vi "check mergeable.vi"(10 "Cube 2":T1, 11 "Cube 1":T1) -> (2 "Merged?":bool, 3 "Cube Out":T1)   [LabVIEW 2021]
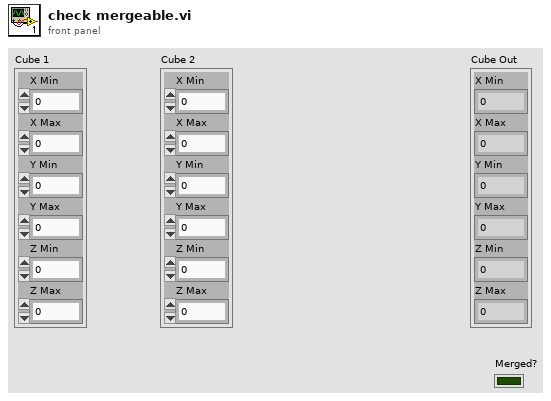
[diagram p1: front panel]
types:
  T1 = cluster{"X Min":i64, "X Max":i64, "Y Min":i64, "Y Max":i64, "Z Min":i64, "Z Max":i64}
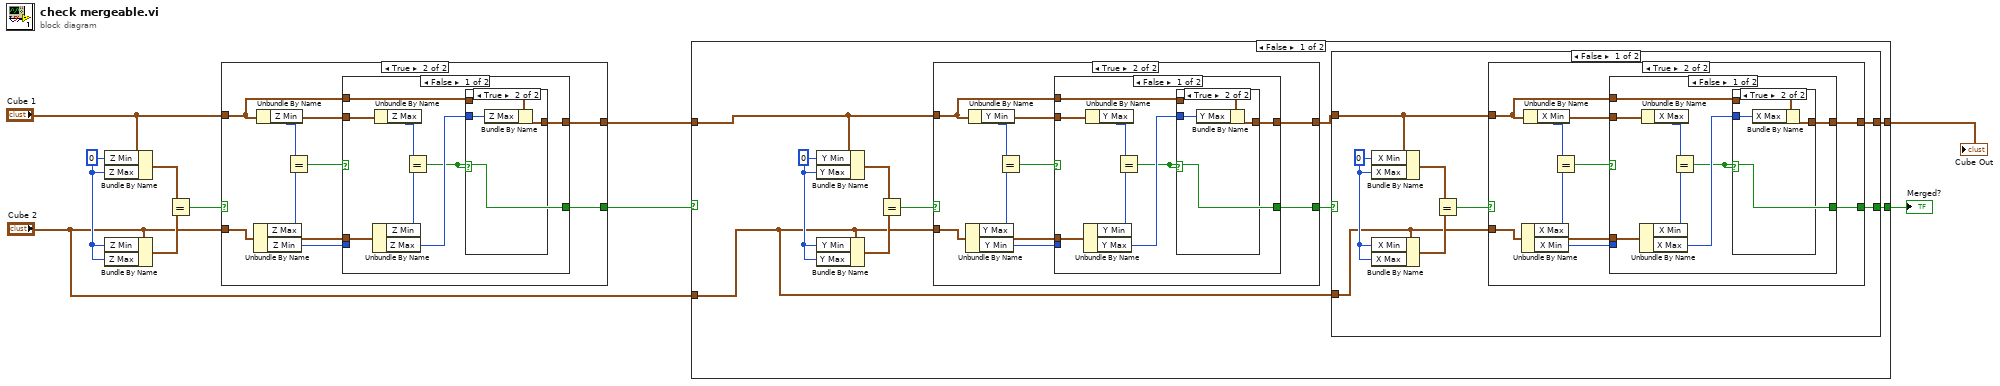
[diagram p0: block diagram]
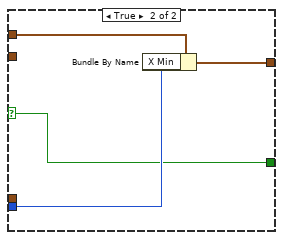
[diagram p4: hidden frame]
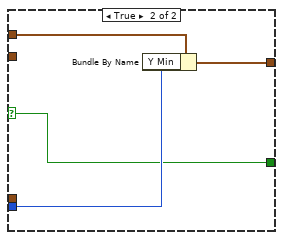
[diagram p8: hidden frame]
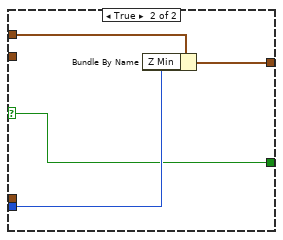
[diagram p12: hidden frame]
diagram:
  w10 = i64 0 ("Z Min")
  n1 = Bundle By Name(cluster="Cube 1", "Z Min"=w10, "Z Max"=w10) -> (w8:T1)
  n2 = Bundle By Name(cluster="Cube 2", "Z Min"=w10, "Z Max"=w10) -> (w9:T1)
  n3 = Equal?(x=w8, y=w9) -> (x = y?=w7:bool)
  n4 = case shown="True" w7 {
    selector: w7 -> [w12 _]
    tunnel: [w12 w15] -> w2
    tunnel: "Cube 1" -> [w11 w13]
    tunnel: "Cube 2" -> [_ w14]
    tunnel: [w11 w17] -> w5
    frame False {
    }
    frame True {
      n5 = Unbundle By Name(w14) -> ("Z Max"=w19:i64, "Z Min"=w18:i64)
      n6 = Unbundle By Name(w13) -> ("Z Min"=w20:i64)
      n7 = Equal?(x=w20, y=w19) -> (x = y?=w16:bool)
      n8 = case shown="False" w16 {
        selector: w16 -> [_ w33]
        tunnel: w13 -> [w24 w36]
        tunnel: w18 -> [_ w35]
        tunnel: [w22 w34] -> w17
        tunnel: [w21 w33] -> w15
        tunnel: w14 -> [w26 _]
        tunnel: w13 -> [w25 _]
        frame False {
          n9 = Unbundle By Name(w26) -> ("Z Min"=w28:i64, "Z Max"=w23:i64)
          n10 = Unbundle By Name(w25) -> ("Z Max"=w27:i64)
          n11 = Equal?(x=w27, y=w28) -> (x = y?=w21:bool)
          n12 = case shown="True" w21 {
            tunnel: w24 -> [w29 w32]
            tunnel: w23 -> [_ w31]
            tunnel: [w29 w30] -> w22
            frame False {
            }
            frame True {
              n13 = Bundle By Name(cluster=w32, "Z Max"=w31) -> (w30:T1)
            }
          }
        }
        frame True {
          n14 = Bundle By Name(cluster=w36, "Z Min"=w35) -> (w34:T1)
        }
      }
    }
  }
  n15 = case shown="False" w2 {
    selector: w2 -> [_ w110]
    tunnel: w5 -> [w42 w109]
    tunnel: "Cube 2" -> [w41 _]
    tunnel: [w39 w110] -> w3
    tunnel: [w37 w109] -> w1
    frame False {
      w43 = i64 0 ("Z Min")
      n16 = Bundle By Name(cluster=w42, "Y Min"=w43, "Y Max"=w43) -> (w45:T1)
      n17 = Bundle By Name(cluster=w41, "Y Min"=w43, "Y Max"=w43) -> (w44:T1)
      n18 = Equal?(x=w45, y=w44) -> (x = y?=w46:bool)
      n19 = case shown="True" w46 {
        selector: w46 -> [w84 _]
        tunnel: [w84 w87] -> w38
        tunnel: w42 -> [w83 w85]
        tunnel: w41 -> [_ w86]
        tunnel: [w83 w89] -> w40
        frame False {
        }
        frame True {
          n20 = Unbundle By Name(w86) -> ("Y Max"=w91:i64, "Y Min"=w90:i64)
          n21 = Unbundle By Name(w85) -> ("Y Min"=w92:i64)
          n22 = Equal?(x=w92, y=w91) -> (x = y?=w88:bool)
          n23 = case shown="False" w88 {
            selector: w88 -> [_ w105]
            tunnel: w85 -> [w96 w108]
            tunnel: w90 -> [_ w107]
            tunnel: [w94 w106] -> w89
            tunnel: [w93 w105] -> w87
            tunnel: w86 -> [w98 _]
            tunnel: w85 -> [w97 _]
            frame False {
              n24 = Unbundle By Name(w98) -> ("Y Min"=w100:i64, "Y Max"=w95:i64)
              n25 = Unbundle By Name(w97) -> ("Y Max"=w99:i64)
              n26 = Equal?(x=w99, y=w100) -> (x = y?=w93:bool)
              n27 = case shown="True" w93 {
                tunnel: w96 -> [w101 w104]
                tunnel: w95 -> [_ w103]
                tunnel: [w101 w102] -> w94
                frame False {
                }
                frame True {
                  n28 = Bundle By Name(cluster=w104, "Y Max"=w103) -> (w102:T1)
                }
              }
            }
            frame True {
              n29 = Bundle By Name(cluster=w108, "Y Min"=w107) -> (w106:T1)
            }
          }
        }
      }
      n30 = case shown="False" w38 {
        selector: w38 -> [_ w82]
        tunnel: w41 -> [w50 _]
        tunnel: w40 -> [w49 w81]
        tunnel: [w48 w82] -> w39
        tunnel: [w47 w81] -> w37
        frame False {
          w54 = i64 0 ("Z Min")
          n31 = Bundle By Name(cluster=w49, "X Min"=w54, "X Max"=w54) -> (w52:T1)
          n32 = Bundle By Name(cluster=w50, "X Min"=w54, "X Max"=w54) -> (w53:T1)
          n33 = Equal?(x=w52, y=w53) -> (x = y?=w51:bool)
          n34 = case shown="True" w51 {
            selector: w51 -> [w56 _]
            tunnel: [w56 w59] -> w48
            tunnel: w49 -> [w55 w57]
            tunnel: w50 -> [_ w58]
            tunnel: [w55 w61] -> w47
            frame False {
            }
            frame True {
              n35 = Unbundle By Name(w58) -> ("X Max"=w63:i64, "X Min"=w62:i64)
              n36 = Unbundle By Name(w57) -> ("X Min"=w64:i64)
              n37 = Equal?(x=w64, y=w63) -> (x = y?=w60:bool)
              n38 = case shown="False" w60 {
                selector: w60 -> [_ w77]
                tunnel: w57 -> [w68 w80]
                tunnel: w62 -> [_ w79]
                tunnel: [w66 w78] -> w61
                tunnel: [w65 w77] -> w59
                tunnel: w58 -> [w70 _]
                tunnel: w57 -> [w69 _]
                frame False {
                  n39 = Unbundle By Name(w70) -> ("X Min"=w72:i64, "X Max"=w67:i64)
                  n40 = Unbundle By Name(w69) -> ("X Max"=w71:i64)
                  n41 = Equal?(x=w71, y=w72) -> (x = y?=w65:bool)
                  n42 = case shown="True" w65 {
                    tunnel: w68 -> [w73 w76]
                    tunnel: w67 -> [_ w75]
                    tunnel: [w73 w74] -> w66
                    frame False {
                    }
                    frame True {
                      n43 = Bundle By Name(cluster=w76, "X Max"=w75) -> (w74:T1)
                    }
                  }
                }
                frame True {
                  n44 = Bundle By Name(cluster=w80, "X Min"=w79) -> (w78:T1)
                }
              }
            }
          }
        }
        frame True {
        }
      }
    }
    frame True {
    }
  }
  "Cube Out" <- w1
  "Merged?" <- w3
